vi "Initialize Panel.vi"(8 "error in (no error)":errorcluster, 11 "vi reference in":refnum<vi>) -> (0 "error out":errorcluster, 2 "initial window state":T1(ring), 3 "vi reference out":refnum<vi>)   [LabVIEW 2019, in "Micron_server.lvlib"]
uses:
  Micron_server.lvlib
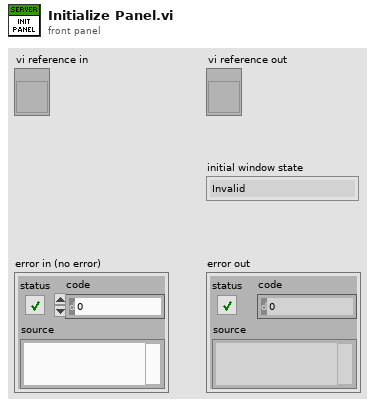
[diagram p1: front panel]
types:
  T1 = enum32{"Invalid", "Standard", "Closed", "Hidden", "Minimized", "Maximized"}
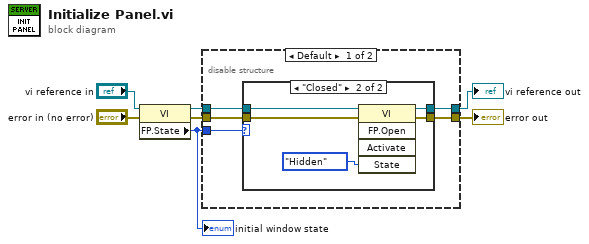
[diagram p0: block diagram]
diagram:
  n1 = property class="VI"(reference="vi reference in", error in="error in (no error)") -> (reference out=w6:refnum<vi>, error out=w5:errorcluster, "FP.State"=w4:T1)
  "initial window state" <- w4
  n2 = disable-structure shown="Default" {
    disable-tunnel: w6 -> [w12 w21]
    disable-tunnel: w5 -> [w11 w20]
    disable-tunnel: w4 -> [w8 _]
    disable-tunnel: [w10 w20] -> w1
    disable-tunnel: [w9 w21] -> w2
    frame condition #0 (active) {
      n3 = case shown="\"Closed\"" w8 {
        tunnel: w12 -> [w14 w18]
        tunnel: w11 -> [w13 w17]
        tunnel: [w13 w16] -> w10
        tunnel: [w14 w15] -> w9
        frame Default {
        }
        frame "Closed" {
          n4 = invoke class="VI" method="FP.Open"(reference=w18, error in=w17, "State"=T1."Hidden") -> (reference out=w15:refnum<vi>, error out=w16:errorcluster)  [unwired: 2 in, 3 out]
        }
      }
    }
    frame condition #1 {
    }
  }
  "vi reference out" <- w2
  "error out" <- w1
